vi "Stop Core.vi"(10 "final error code":i32, 11 "Elevator Controller in":refnum<class "Elevator Controller.lvclass">) -> (3 "Elevator Controller out":refnum<class "Elevator Controller.lvclass">)   [LabVIEW 2019, in "Elevator Controller Actor.lvlib" / "Elevator Controller.lvclass"]
doc: "(<B>Filename</B>: Actor Framework.lvlib:Actor.lvclass:Stop Core.vi)\n\nDefines what the actor does before it stops. Use the <B>final error code</B> input to determine whether the actor shut down in response to an error.\n\nBy default, this method passes the Stop message along to all auto-stop nested actors. A descendant class may override this method to define additional behavior, such as shutting down any processes the actor initiated in its override of the Actor Core method."
uses:
  Elevator Controller.lvclass
  Elevator Controller.lvclass/Elevator Controller.ctl
  <vilib>/ActorFramework/Actor/Actor.lvclass
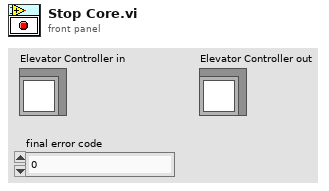
[diagram p1: front panel]
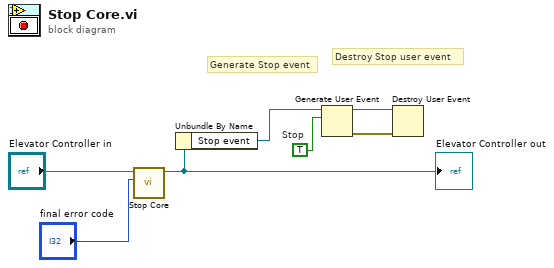
[diagram p0: block diagram]
diagram:
  w1 = TRUE  # Stop
  # "Destroy Stop user event"
  # "Generate Stop event"
  n1 = call-parent "Stop Core.vi"("final error code"="final error code", "Actor in"="Elevator Controller in") -> ("Actor out"=w5:refnum<class "Elevator Controller.lvclass">)  [unwired: 9 in]
  "Elevator Controller out" <- w5
  n2 = Unbundle By Name(w5) -> ("Stop event"=w4:refnum<user-event>)
  n3 = Generate User Event(user event=w4, event data cluster=w1) -> (user event out=w2:refnum<user-event>, error out=w3:errorcluster)  [unwired: 2 in]
  n4 = Destroy User Event(user event=w2, error in=w3) -> ()  [unwired: 1 out]
